vi "AprilTag Slice Testing.vi"(1 "Detector Settings":T5={"Refine Edges (Default: True)"=FALSE, "Threads (Default: 1)"=3, "Decimate (Default: 1)"=1.0, "Blur (Default: 0)"=0.0, "Bits (Default: 2)"=2} {"Threads (Default: 1)" min=1}, 5 "Greyscale Image":T1, 7 "Display":bool, 9 "slices":i32=1, 11 "dbg index":i32) -> (3 "Greyscale Image 2":T1, 4 "Detections":T2[](array[typedef]), 6 "gray":dbl, 8 "2D Picture 2":picture, 10 "detect":dbl, 15 "2D Picture":picture)   [LabVIEW 2025]
uses:
  <vilib>/Serenial/G Augmented-Reality Toolkit/g_ar_toolkit.common/Image Size (Integer).ctl
  <vilib>/Serenial/G Augmented-Reality Toolkit/g_ar_toolkit.feature_detection/Apriltag Detector/Detector Settings.ctl
  <vilib>/Serenial/G Augmented-Reality Toolkit/g_ar_toolkit.common/Image Point (Float).ctl
  <vilib>/Serenial/G Augmented-Reality Toolkit/g_ar_toolkit.feature_detection/Apriltag Detector/Detection.ctl
  <vilib>/Serenial/G Augmented-Reality Toolkit/g_ar_toolkit.common/Quad Corners.ctl
  <vilib>/Serenial/G Augmented-Reality Toolkit/g_ar_toolkit.image/Greyscale Image.ctl
  <vilib>/Serenial/G Augmented-Reality Toolkit/g_ar_toolkit.feature_detection/Apriltag Detector/AprilTag Detector.lvclass/AprilTag Detector.ctl
  9e7906d5-2bde-47e0-b1aa-b96b80dd5951.vi
  a86f0687-08f4-4781-acff-0da3162c1161.vi
  <vilib>/Serenial/G Augmented-Reality Toolkit/g_ar_toolkit.feature_detection/Apriltag Detector/Create (Tag36h11).vi
  <vilib>/Serenial/G Augmented-Reality Toolkit/g_ar_toolkit.image/Size (Greyscale).vi
  <vilib>/Serenial/G Augmented-Reality Toolkit/g_ar_toolkit.image/Draw Image to Picture (Greyscale).vi
  <vilib>/Serenial/G Augmented-Reality Toolkit/g_ar_toolkit.common/NI-Linux-RT Shared Library Path (Feature Detection).vi
  <vilib>/Serenial/G Augmented-Reality Toolkit/g_ar_toolkit.common/NI-Linux-RT Shared Library Path (Core).vi
  <vilib>/Serenial/G Augmented-Reality Toolkit/g_ar_toolkit.common/NI-Linux-RT Shared Library Path.vi
  <vilib>/Serenial/G Augmented-Reality Toolkit/g_ar_toolkit.feature_detection/Apriltag Detector/CreateDetector.vi
  <vilib>/Utility/error.llb/Error Cluster From Error Code.vi
  <vilib>/Serenial/G Augmented-Reality Toolkit/g_ar_toolkit.image/g_ar_toolkit.image.lvlib
  <vilib>/Serenial/G Augmented-Reality Toolkit/g_ar_toolkit.feature_detection/Apriltag Detector/AprilTag Detector.lvclass
  <vilib>/Serenial/G Augmented-Reality Toolkit/g_ar_toolkit.common/g_ar_toolkit.common.lvlib
panel:
  in  "color":u32(colorbox)=16722479
  in  "Poly":bool
  out "size(s)":i32
  in  "overlap":i32=200
  in  "origin":T3={"x"=0.0, "y"=400.0}
  in  "size":T6={"Width"=2880, "Height"=900}
  out "good tag details":T7(array[cluster])
  # "Angles between\ntarget and camera"
  # "Offset between\ntarget and camera"
  # "Better way to pick camera matrix\ncheck other cams and simplify scaling"
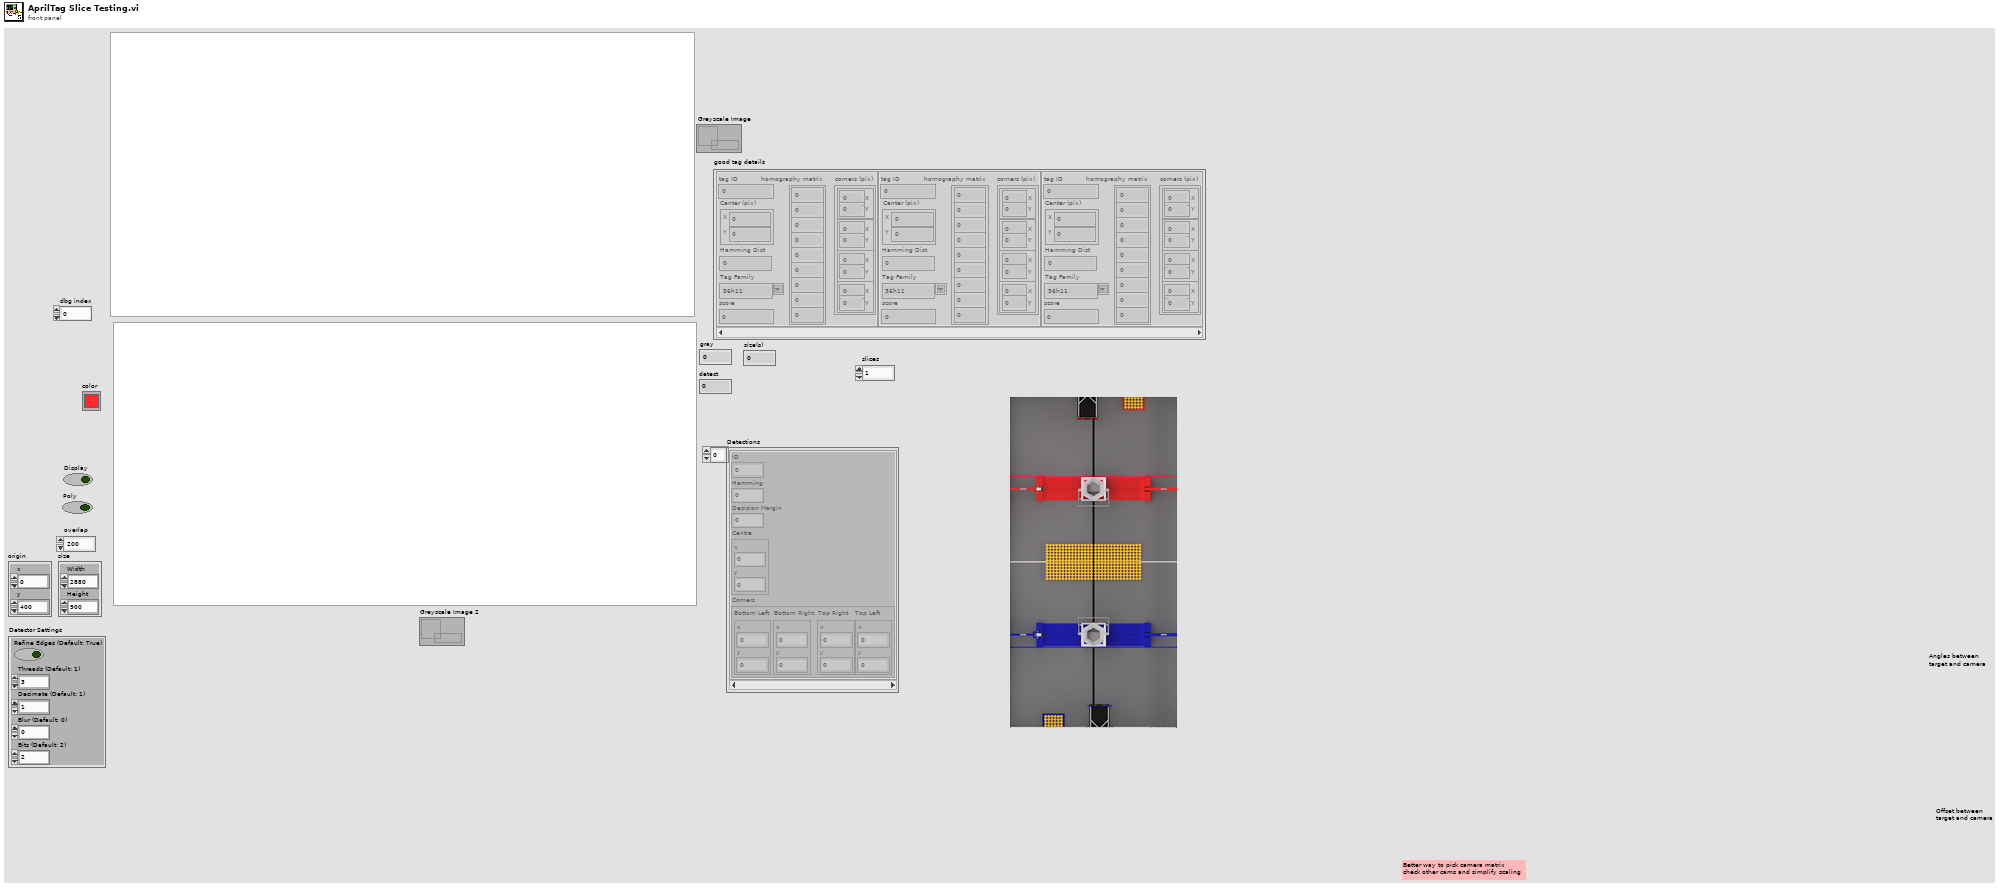
[diagram p1: front panel]
types:
  T1 = typedef "g_ar_toolkit.image.lvlib/Greyscale Image.ctl" = refnum<data-value>
  T2 = typedef "g_ar_toolkit.feature_detection.lvlib/AprilTag Detector.lvclass/Detection.ctl" = cluster{"ID":i32, "Hamming":i32, "Decision Margin":sgl, "Centre":T3, "Corners":T4}
  T3 = typedef "g_ar_toolkit.common.lvlib/Image Point (Float).ctl" = cluster{"x":dbl, "y":dbl}
  T4 = typedef "g_ar_toolkit.common.lvlib/Quad Corners.ctl" = cluster{"Bottom Left":T3, "Bottom Right":T3, "Top Right":T3, "Top Left":T3}
  T5 = typedef "g_ar_toolkit.feature_detection.lvlib/AprilTag Detector.lvclass/Detector Settings.ctl" = cluster{"Refine Edges (Default: True)":bool, "Threads (Default: 1)":u8, "Decimate (Default: 1)":sgl, "Blur (Default: 0)":sgl, "Bits (Default: 2)":u8}
  T6 = typedef "g_ar_toolkit.common.lvlib/Image Size (Integer).ctl" = cluster{"Width":u16, "Height":u16}
  T7 = cluster{"tag ID":i32, "Center (pix)":cluster{"X":dbl, "Y":dbl}, "homography matrix":dbl[], "score":dbl, "Hamming Dist":i32, "corners (pix)":cluster{"X":dbl, "Y":dbl}[], "Tag Family":string}[]
  T8 = cluster{"size":T6, "origin":T3, "overlap":i32, "slices":i32}
  T9 = cluster{"size":cluster{"Width":dbl, "height":dbl}, "offset":cluster{"x":dbl, "y":dbl}}[]
  T10 = cluster{"size":cluster{"Width":dbl, "height":dbl}, "offset":cluster{"x":dbl, "y":dbl}}
  T11 = cluster{"tag ID":i32, "Center":cluster{"X":dbl, "Y":dbl}, "Homography Matrix":dbl[], "dec margin":dbl, "Hamming Dist":i32, "Corner Points":cluster{"X":dbl, "Y":dbl}[], "Tag Family":string}[]
  T12 = cluster{"Width":u16, "Style":enum32{"Solid", "Dash", "Dot", "DashDot", "DashDotDot"}}
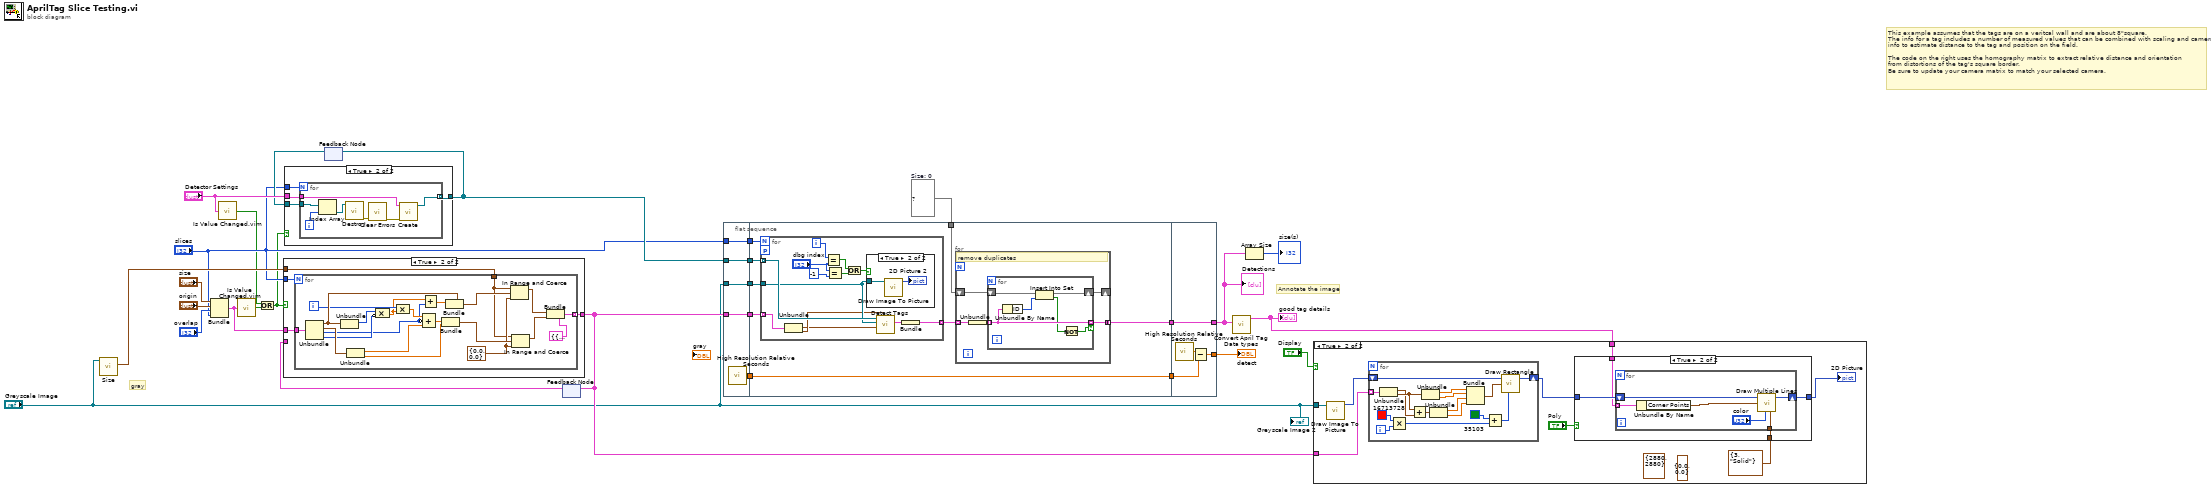
[diagram p0: block diagram]
diagram:
  w2 = set{i32} {}  # Size: 0
  # "Annotate the image"
  # "gray"
  # "This example assumes that the tags are on a veritcal wall and are about 8\"square. \nThe info for a tag includes a number of measured values that can be combined with scaling and camera\ninfo to estimate distance to the tag and position on the field. \n\nThe code on the right uses the homography matrix to extract relative distance and orientation\nfrom distortions of the tag's square border.\nBe sure to update your camera matrix to match your selected camera."
  n1 = call-poly <vilib>:"Size.vi"("Greyscale Image in"="Greyscale Image") -> ("Image Size"=w28:T6)  [unwired: 8 in, 2 out]
  n2 = Bundle("size"="size", "origin"="origin", "overlap"="overlap", "slices"="slices") -> (w14:T8)  [unwired: 1 in]
  n3 = call "Is Value Changed.vim"("value"="Detector Settings") -> ("changed or first call?"=w8:bool)
  n4 = call "Is Value Changed.vim"("value"=w14) -> ("changed or first call?"=w10:bool)
  n5 = Or(x=w8, y=w10) -> (x .or. y?=w9:bool)
  n6 = feedback #1() -> (w18:refnum<class "AprilTag Detector.lvclass">[])  [unwired: 1 in]
  n7 = case shown="True" w9 {
    tunnel: [w29 w33] -> w13
    tunnel: "Detector Settings" -> [_ w31]
    tunnel: w18 -> [w29 w32]
    tunnel: "slices" -> [_ w30]
    frame False {
    }
    frame True {
      n8 = for {
        N: w30 -> [_]
        tunnel: [w40] -> w33 mode=indexing
        tunnel: w32 -> [w35]
        tunnel: w31 -> [w37]
        i -> [w36]
        n9 = Index Array(array=w35, index=w36) -> (element=w34:refnum<class "AprilTag Detector.lvclass">)
        n10 = call <vilib>:"Destroy.vi"("Apriltag Detector in"=w34) -> ("error out"=w39:errorcluster)  [unwired: 10 in]
        n11 = call <vilib>:"Clear Errors.vi"("error in (no error)"=w39) -> ("error out"=w38:errorcluster)  [unwired: 5 in, 1 out]
        n12 = call-poly <vilib>:"Create.vi"("error in (no error)"=w38, "Detector Settings"=w37) -> ("Apriltag Detector"=w40:refnum<class "AprilTag Detector.lvclass">)  [unwired: 8 in, 1 out]
      }
    }
  }
  n13 = feedback-in #1(w13) -> ()
  n14 = feedback #2() -> (w7:T9)  [unwired: 1 in]
  n15 = case shown="True" w9 {
    tunnel: [w41 w45] -> w4
    tunnel: w14 -> [_ w43]
    tunnel: "slices" -> [_ w44]
    tunnel: w7 -> [w41 _]
    tunnel: w28 -> [_ w42]
    frame False {
    }
    frame True {
      n16 = for {
        N: w44 -> [_]
        tunnel: [w60] -> w45 mode=indexing
        tunnel: w43 -> [w59]
        tunnel: w42 -> [w47]
        i -> [w56]
        w48 = cluster{dbl, "y":dbl} {0.0, "y"=0.0} ("lower limit")
        n17 = Unbundle(w59) -> ("size"=w63:T6, "origin"=w65:T3, "overlap"=w53:i32, "slices"=w58:i32)
        n18 = Unbundle(w63) -> ("Width"=w66:u16)  [unwired: 1 out]
        n19 = Unbundle(w65) -> ("x"=w64:dbl, "y"=w61:dbl)
        n20 = Compound Arithmetic op=MULTIPLY(w66, invert w58) -> (w54:dbl)
        n21 = Compound Arithmetic op=MULTIPLY(w56, w54) -> (w57:dbl)
        n22 = Add(x=w54, y=w53) -> (x+y=w55:dbl)
        n23 = Compound Arithmetic op=ADD(w57, invert w53, w64) -> (w62:dbl)
        n24 = Bundle(w62, "y"=w61) -> (w52:cluster{dbl, "y":dbl})  [unwired: 1 in]
        n25 = Bundle(cluster=w63, "Width"=w55) -> (w51:T6)  [unwired: 1 in]
        n26 = In Range and Coerce(upper limit=w47, x=w51, lower limit=w48) -> (coerced(x)=w49:cluster{"Width":dbl, "y":dbl})  [unwired: 1 out]
        n27 = In Range and Coerce(upper limit=w47, x=w52, lower limit=w48) -> (coerced(x)=w50:cluster{"Width":dbl, "y":dbl})  [unwired: 1 out]
        n28 = Bundle(cluster=T10 {"size"={"Width"=0.0, "height"=0.0}, "offset"={"x"=0.0, "y"=0.0}}, "size"=w49, "offset"=w50) -> (w60:T10)
      }
    }
  }
  n29 = feedback-in #2(w4) -> ()
  n30 = flat-sequence {
    tunnel: "slices" -> [w68]
    tunnel: "Greyscale Image" -> [w69]
    tunnel: w13 -> [w70]
    tunnel: w4 -> [w71]
    tunnel: [w71] -> w27
    tunnel: [w70] -> w26
    tunnel: [w69] -> w25
    tunnel: [w68] -> w24
    tunnel: [w67] -> w23
    tunnel: [w73] -> w22
    tunnel: w27 -> [w74]
    tunnel: w26 -> [w78]
    tunnel: w25 -> [w77]
    tunnel: w24 -> [w76]
    tunnel: [w75] -> w21
    tunnel: w23 -> [w75]
    tunnel: w2 -> [w72]
    tunnel: [w109] -> w6
    tunnel: w22 -> [w109]
    tunnel: w21 -> [w108]
    tunnel: [w106] -> w11
    frame #0 {
      n31 = call <vilib>:"High Resolution Relative Seconds.vi"() -> ("relative seconds"=w67:dbl)
    }
    frame #1 {
      n32 = for {
        N: w76 -> [_]
        tunnel: w74 -> [w93] mode=indexing
        tunnel: w77 -> [w94]
        tunnel: w78 -> [w103] mode=indexing
        tunnel: [w102] -> w79 mode=indexing
        workers-P: _ -> [_]
        i -> [w100]
        n33 = Unbundle(w93) -> ("size"=w91:cluster{"Width":dbl, "height":dbl}, "offset"=w92:cluster{"x":dbl, "y":dbl})
        n34 = Equal?(x=w100, y="dbg index") -> (x = y?=w96:bool)
        n35 = Equal?(x="dbg index", y=-1) -> (x = y?=w95:bool)
        n36 = Or(x=w96, y=w95) -> (x .or. y?=w97:bool)
        n37 = case shown="True" w97 {
          tunnel: w94 -> [_ w105]
          frame False {
          }
          frame True {
            n38 = call-poly <vilib>:"Draw Image To Picture.vi"("Greyscale Image Source in"=w105) -> ("Picture"=→"2D Picture 2":picture)  [unwired: 9 in, 1 out]
          }
        }
        n39 = call <vilib>:"Detect Tags.vi"("Region Offset (Default: 0,0)"=w92, "Region Size (Default:0,0 - Whole Image)"=w91, "Greyscale Image in"=w94, "Apriltag Detector in"=w103) -> ("Detections"=w101:T2[])  [unwired: 3 in, 4 out]
        n40 = Bundle("Detections"=w101) -> (w102:cluster{"Detections":T2[]})  [unwired: 1 in]
      }
      n41 = for {
        tunnel: w79 -> [w84] mode=indexing
        tunnel: [w80] -> w73 mode=concatenating
        shift-right: [w81] -> _
        shift-left: w72 -> [w82]
        # "remove duplicates"
        n42 = Unbundle(w84) -> ("Detections"=w83:T2[])
        n43 = for {
          tunnel: w83 -> [w87] mode=indexing
          shift-right: [w88] -> w81
          shift-left: w82 -> [w89]
          tunnel: [w87] -> w80 mode=indexing if=w85
          n44 = Unbundle By Name(w87) -> ("ID"=w90:i32)
          n45 = Insert Into Set(10:w90, 11:w89) -> (2:w86:bool, 3:w88:set{i32})
          n46 = Not(x=w86) -> (.not. x?=w85:bool)
        }
      }
    }
    frame #2 {
      n47 = call <vilib>:"High Resolution Relative Seconds.vi"() -> ("relative seconds"=w107:dbl)
      n48 = Subtract(x=w107, y=w108) -> (x-y=w106:dbl)
    }
  }
  n49 = call "Convert April Tag Data types.vi"("Detections in"=w6) -> ("tags"=w3:T11)  [unwired: 10 in]
  "good tag details" <- w3
  n50 = Array Size(array=w6) -> (size(s)=→"size(s)":i32)
  n51 = case shown="True" "Display" {
    tunnel: "Greyscale Image" -> [_ w117]
    tunnel: w4 -> [_ w115]
    tunnel: w3 -> [_ w113]
    frame False {
    }
    frame True {
      (unwired) cluster{"X":i32, "Y":i32} {"X"=2880, "Y"=2880} ("Point Coordinates")
      (unwired) cluster{"X":dbl, "Y":dbl} {"X"=0.0, "Y"=0.0} ("Point Coordinates")
      n52 = call-poly <vilib>:"Draw Image To Picture.vi"("Greyscale Image Source in"=w117) -> ("Picture"=w116:picture)  [unwired: 9 in, 1 out]
      n53 = for {
        shift-right: [w143] -> w112
        shift-left: w116 -> [w144]
        tunnel: w115 -> [w129] mode=indexing
        i -> [w134]
        n54 = Unbundle(w129) -> ("size"=w139:cluster{"Width":dbl, "height":dbl}, "offset"=w140:cluster{"x":dbl, "y":dbl})
        n55 = Multiply(x=u32 16713728 ("color(black)"), y=w134) -> (x*y=w132:u32)
        n56 = Add(x=w140, y=w139) -> (x+y=w138:cluster{dbl, dbl})
        n57 = Unbundle(w140) -> ("x"=w142:dbl, "y"=w141:dbl)
        n58 = Unbundle(w138) -> (w137:dbl, w136:dbl)
        n59 = Bundle("x"=w142, "y"=w141, w137, w136) -> (w135:cluster{"x":dbl, "y":dbl, dbl, dbl})  [unwired: 1 in]
        n60 = Add(x=u32 35103 ("color(black)"), y=w132) -> (x+y=w131:u32)
        n61 = call <vilib>:"Draw Rectangle.vi"("picture"=w144, "rect"=w135, "color(black)"=w131) -> ("new picture"=w143:picture)  [unwired: 6 in]
      }
      n62 = case shown="True" "Poly" {
        tunnel: w112 -> [w118 w122]
        tunnel: [w118 w121] -> w111
        tunnel: w113 -> [_ w120]
        tunnel: T12 {"Width"=3, "Style"=enum."Solid"} ("pen") -> [_ w119]
        frame False {
        }
        frame True {
          n63 = for {
            shift-right: [w126] -> w121
            shift-left: w122 -> [w127]
            tunnel: w120 -> [w128] mode=indexing
            tunnel: w119 -> [w124]
            n64 = Unbundle By Name(w128) -> ("Corner Points"=w123:cluster{"X":dbl, "Y":dbl}[])
            n65 = call <vilib>:"Draw Multiple Lines.vi"("picture"=w127, "line endpoints"=w123, "color(black)"="color", "pen"=w124) -> ("new picture"=w126:picture)  [unwired: 5 in]
          }
        }
      }
      "2D Picture" <- w111
    }
  }
  "detect" <- w11
  "Detections" <- w6
  "Greyscale Image 2" <- "Greyscale Image"
